vi "Logout User.vi"(8 "error in (no error)":errorcluster) -> (0 "error out":errorcluster)   [LabVIEW 2019]
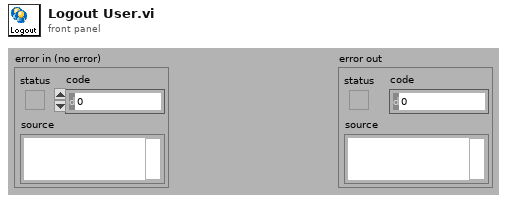
[diagram p1: front panel]
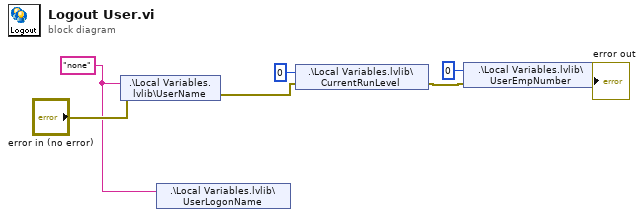
[diagram p0: block diagram]
diagram:
  w1 = "none" ("UserName")
  n1 = shared-variable ".\\Local Variables.lvlib\\UserName"(w1, error in="error in (no error)") -> (error out=w4:errorcluster)
  n2 = shared-variable ".\\Local Variables.lvlib\\UserLogonName"(w1) -> ()  [unwired: 1 in, 1 out]
  n3 = shared-variable ".\\Local Variables.lvlib\\CurrentRunLevel"(0 ("CurrentRunLevel"), error in=w4) -> (error out=w3:errorcluster)
  n4 = shared-variable ".\\Local Variables.lvlib\\UserEmpNumber"(0 ("UserEmpNumber"), error in=w3) -> (error out=→"error out":errorcluster)
